vi "ExtractINIInfo.vi"(11 "INI File Path":path) -> (1 "Plugin Name":string, 2 "Instrument Class Path":path, 3 "INI Info":T1)   [LabVIEW 2018]
uses:
  TypeDefs/INIInfo.ctl
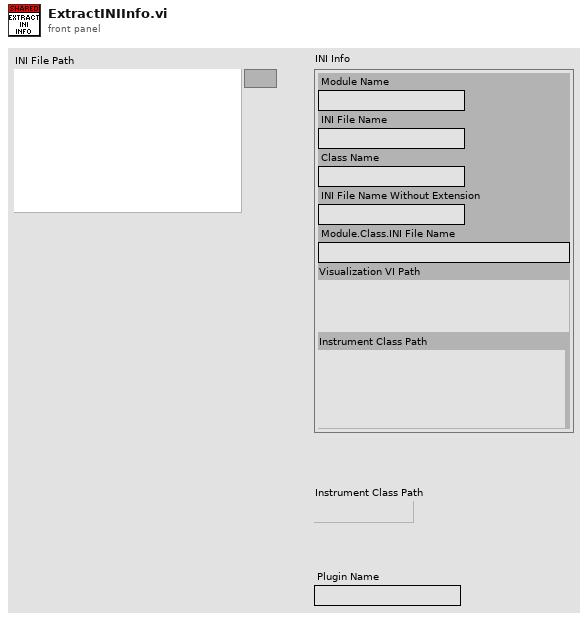
[diagram p1: front panel]
types:
  T1 = typedef "INIInfo.ctl" = cluster{"Module Name":string, "INI File Name":string, "Class Name":string, "INI File Name Without Extension":string, "Module.Class.INI File Name":string, "Visualization VI Path":path, "Instrument Class Path":path}
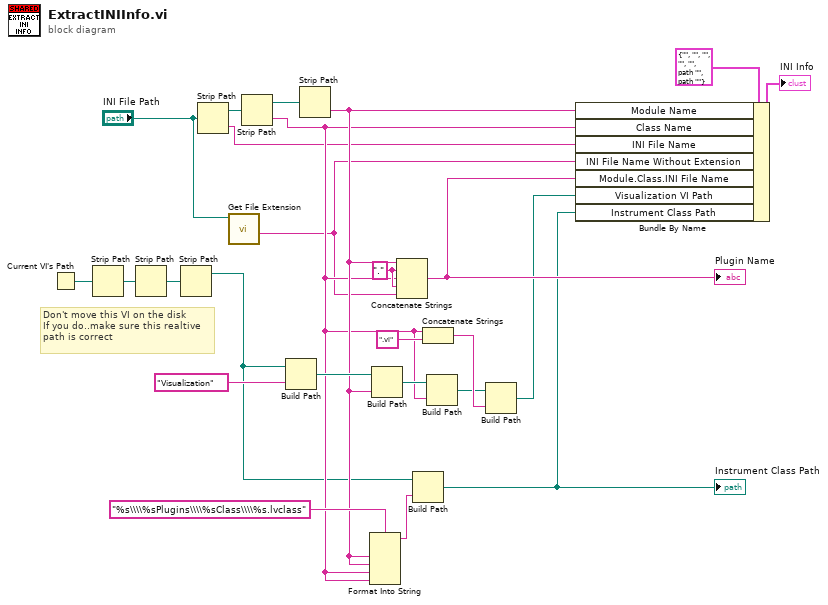
[diagram p0: block diagram]
diagram:
  w16 = "." ("string")
  # "Don't move this VI on the disk\nIf you do..make sure this realtive\npath is correct"
  n1 = Current VI's Path() -> (path=w4:path)
  n2 = Strip Path(path=w4) -> (stripped path=w3:path)  [unwired: 1 out]
  n3 = Strip Path(path=w3) -> (stripped path=w2:path)  [unwired: 1 out]
  n4 = Strip Path(path=w2) -> (stripped path=w1:path)  [unwired: 1 out]
  n5 = Strip Path(path="INI File Path") -> (stripped path=w24:path, name=w9:string)
  n6 = call <vilib>:"Get File Extension.vi"("file"="INI File Path") -> ("filename without extension"=w8:string)  [unwired: 6 in, 4 out]
  n7 = Strip Path(path=w24) -> (stripped path=w25:path, name=w10:string)
  n8 = Build Path(base path=w1, name or relative path="Visualization") -> (appended path=w21:path)
  n9 = Strip Path(path=w25) -> (name=w11:string)  [unwired: 1 out]
  n10 = Format Into String(format string="%s\\\\%sPlugins\\\\%sClass\\\\%s.lvclass" ("name or relative path"), w11, w11, w10, w10) -> (resulting string=w17:string)  [unwired: 2 in, 1 out]
  n11 = Build Path(base path=w21, name or relative path=w11) -> (appended path=w15:path)
  n12 = Concatenate Strings(w11, w16, w10, w16, w8) -> (w7:string)
  "Plugin Name" <- w7
  n13 = Build Path(base path=w1, name or relative path=w17) -> (appended path=w5:path)
  "Instrument Class Path" <- w5
  n14 = Concatenate Strings(w10, ".vi" ("string")) -> (w20:string)
  n15 = Build Path(base path=w15, name or relative path=w10) -> (appended path=w14:path)
  n16 = Build Path(base path=w14, name or relative path=w20) -> (appended path=w6:path)
  n17 = Bundle By Name(cluster=T1 {"Module Name"="", "INI File Name"="", "Class Name"="", "INI File Name Without Extension"="", "Module.Class.INI File Name"="", "Visualization VI Path"=path "", "Instrument Class Path"=path ""} ("INI Info"), "Module Name"=w11, "Class Name"=w10, "INI File Name"=w9, "INI File Name Without Extension"=w8, "Module.Class.INI File Name"=w7, "Visualization VI Path"=w6, "Instrument Class Path"=w5) -> (→"INI Info":T1)
